vi "build.proc.vi"(8 "error in":errorcluster, 10 "Flow":T1[](array[typedef]), 11 "Proc Head":T3={"Procedure Name"="MyProcExample", "Running"=TRUE, "tags"="MyProcExample"}) -> (0 "error out":errorcluster, 3 "Instructions":variant[](array[variant]))   [LabVIEW 2024]
uses:
  controls/UiProcHeader.ctl
  controls/UiStepBuilder.ctl
  controls/type.step-builder.ctl
  build.flowToVarient.vi
  Polymorphics/variantCtrl.polymorphic.vi
  Polymorphics/variantCtrlStepFunction.vi
  Polymorphics/variantCtrlSetpoint.vi
  Polymorphics/variantCtrlString.vi
  proc.util.enumToStrStepVar.vi
  util.DelimitedStringFromArray.vi
  Polymorphics/variantCtrlNumber.vi
  util.DelimitedStringToArray.vi
  proc.util.validateParamExist.vi
  <vilib>/Utility/error.llb/Clear Errors.vi
  <vilib>/Utility/error.llb/Trim Whitespace.vi
  <vilib>/Utility/error.llb/Trim Whitespace One-Sided.vi
  build.elementToParamString.vi
  util.error.create.vi
  Polymorphics/variantCtrlStepPointer.vi
  Polymorphics/variantCtrlStepUserMessage.vi
  Polymorphics/variantCtrlStepPath.vi
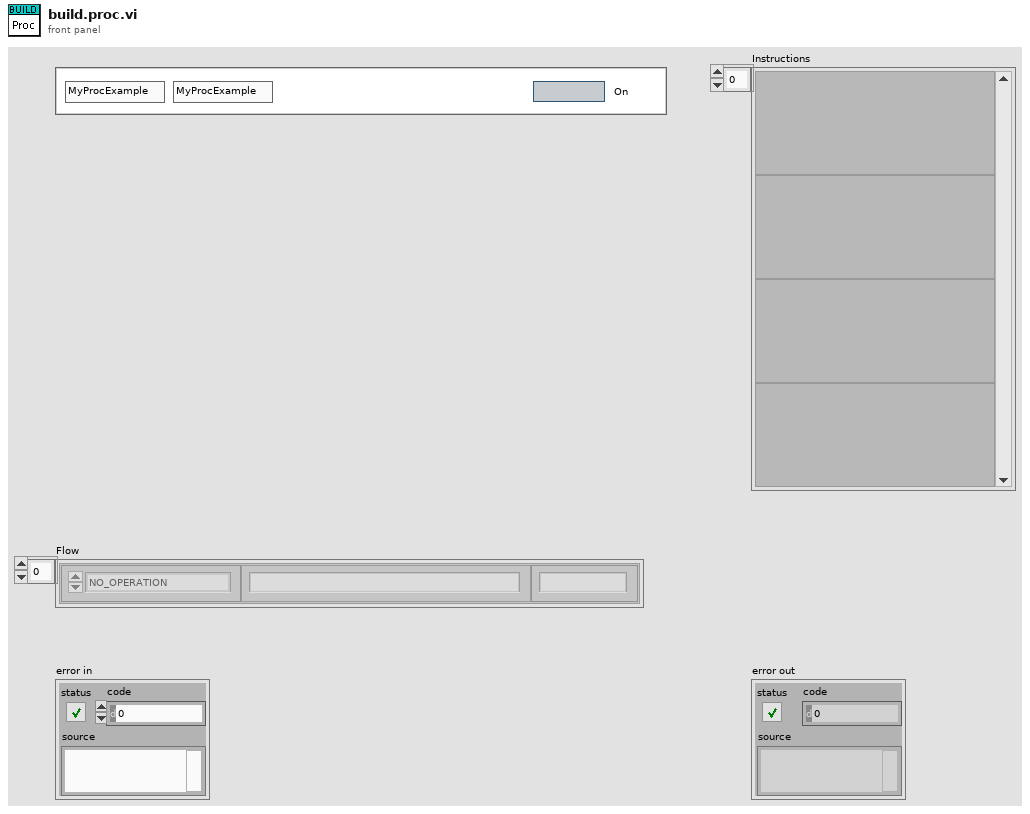
[diagram p1: front panel]
types:
  T1 = typedef "UiStepBuilder.ctl" = cluster{"Step Function":T2, "ParamString":string, "Step Label":string}
  T2 = typedef "type.step-builder.ctl" = enum16{"NO_OPERATION", "DELAY-JUMP", "DELAY", "JUMP", "COMPLETE", "SCHEDULER", "IRR-CHECK", "UNIT-CHECK", "UNIT-SAMPLE", "UNIT-DOSE", "LOG-REPORT", "LOG-MESSAGE", "IO-READ", "IO-READ-MANY", "IO-WRITE", "IO-COMPARE-OUT", "IO-COMPARE-IN", "PROC-START", "PROC-STOP", "PROC-LOAD", "PROC-IS-COMPLETED", "RECORD-MOVE", "GET-RH", "GET-UV", "GET-WD", "GET-WS", "OCS-CHECK", "OCS-RECORD"}
  T3 = typedef "UiProcHeader.ctl" = cluster{"Procedure Name":string, "Running":bool, "tags":string}
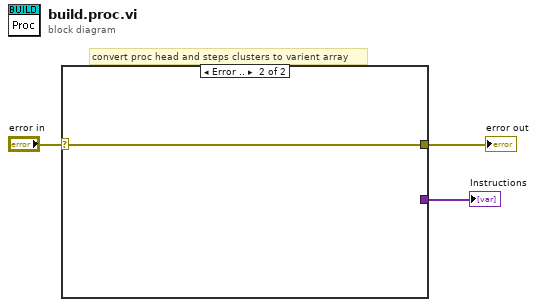
[diagram p0: block diagram]
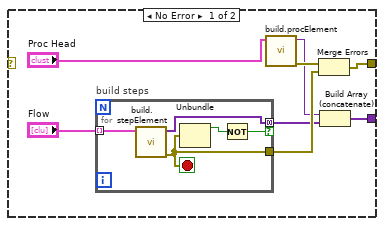
[diagram p2: hidden frame]
diagram:
  # "convert proc head and steps clusters to varient array"
  n1 = case shown="Error .." "error in" {
    selector: "error in" -> [_ w17]
    tunnel: [w10 w17] -> w3
    tunnel: [w8 _] -> w2
    frame No Error {
      n2 = for "build steps" {
        tunnel: "Flow" -> [w12] mode=indexing
        tunnel: [w16] -> w6 mode=concatenating if=w13
        tunnel: [w15] -> w11
        stop <- w15 stop-if-true
        n3 = call "build.stepElement.vi"("Step in"=w12) -> ("error out"=w15:errorcluster, "steps out"=w16:variant[])  [unwired: 9 in]
        n4 = Unbundle(w15) -> ("status"=w14:bool)  [unwired: 2 out]
        n5 = Not(x=w14) -> (.not. x?=w13:bool)
      }
      n6 = call "build.procElement.vi"("UiBuildProcHead"="Proc Head") -> ("error out"=w9:errorcluster, "procElement out"=w7:variant)  [unwired: 9 in]
      n7 = Merge Errors(w9, w11) -> (w10:errorcluster)
      n8 = Build Array (concatenate)(w7, w6) -> (w8:variant[])
    }
    frame Error {
    }
  }
  "Instructions" <- w2
  "error out" <- w3
